vi "dobuncho.vi"(11 "Numeric in":dbl) -> (1 "Numeric out":dbl, 2 "String":string, 3 "String 2":string)   [LabVIEW 2020]
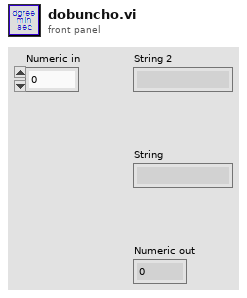
[diagram p1: front panel]
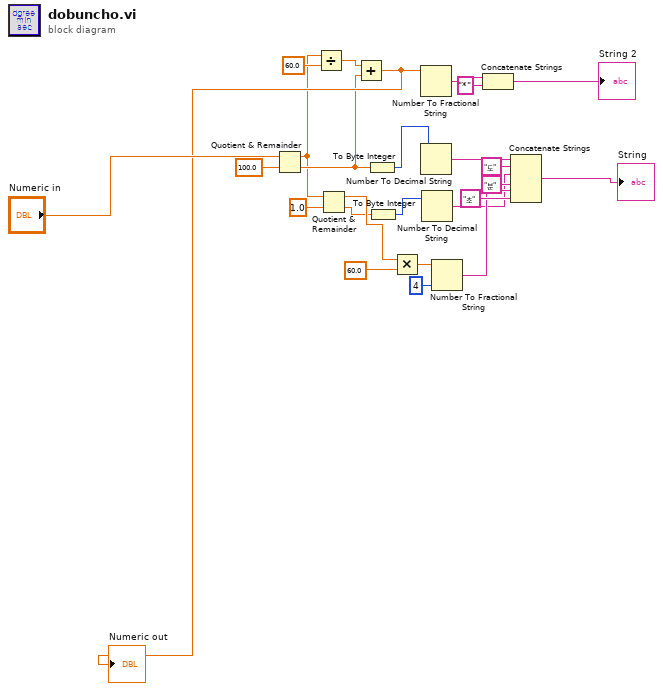
[diagram p0: block diagram]
diagram:
  n1 = Quotient & Remainder(x="Numeric in", y=100.0) -> (x-y*floor(x/y)=w2:dbl, floor(x/y)=w9:dbl)
  n2 = Divide(x=w2, y=60.0) -> (x/y=w4:dbl)
  n3 = Quotient & Remainder(x=w2, y=1.0) -> (x-y*floor(x/y)=w13:dbl, floor(x/y)=w12:dbl)
  n4 = Add(x=w4, y=w9) -> (x+y=w24:dbl)
  "Numeric out" <- w24
  n5 = To Byte Integer(number=w9) -> (8bit integer=w10:i8)
  n6 = To Byte Integer(number=w12) -> (8bit integer=w11:i8)
  n7 = Multiply(x=w13, y=60.0) -> (x*y=w15:dbl)
  n8 = Number To Fractional String(number=w24) -> (F-format string=w6:string)  [unwired: 3 in]
  n9 = Number To Decimal String(number=w10) -> (decimal integer string=w17:string)  [unwired: 1 in]
  n10 = Number To Decimal String(number=w11) -> (decimal integer string=w19:string)  [unwired: 1 in]
  n11 = Number To Fractional String(number=w15, precision (6)=i16 4) -> (F-format string=w21:string)  [unwired: 2 in]
  n12 = Concatenate Strings(w6, "*" ("string")) -> (→"String 2":string)
  n13 = Concatenate Strings(w17, "도" ("string"), w19, "분" ("string"), w21, "초" ("string")) -> (→"String":string)
